vi "Teleop - Motor Data Logger (SubVI).vi"(4 "% Output":dbl, 6 "Battery Voltage":dbl, 7 "Reset":bool, 8 "Current":dbl, 10 "Velocity (ticks/100ms)":dbl, 11 "Position (ticks)":dbl) -> (0 "was teleop?":bool=TRUE, 1 "Time                            Position                    Velocity (RPM)          Acceleration             Current                     % Output                 Battery Voltage":dbl[][](array[numeric]), 2 "Delta V":dbl, 3 "acceleration":u32)   [LabVIEW 2019]
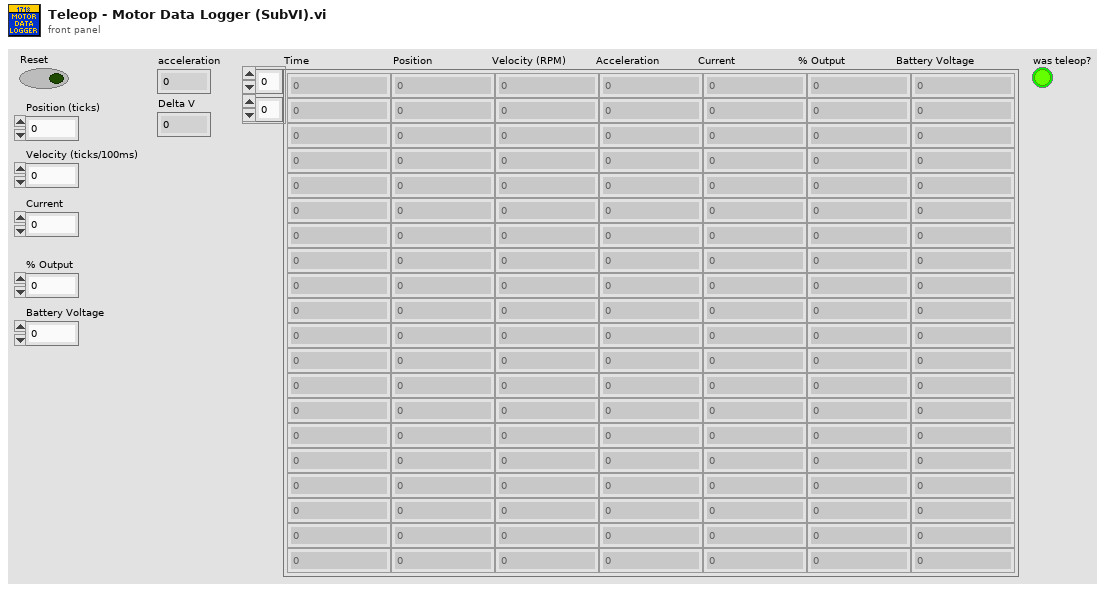
[diagram p1: front panel]
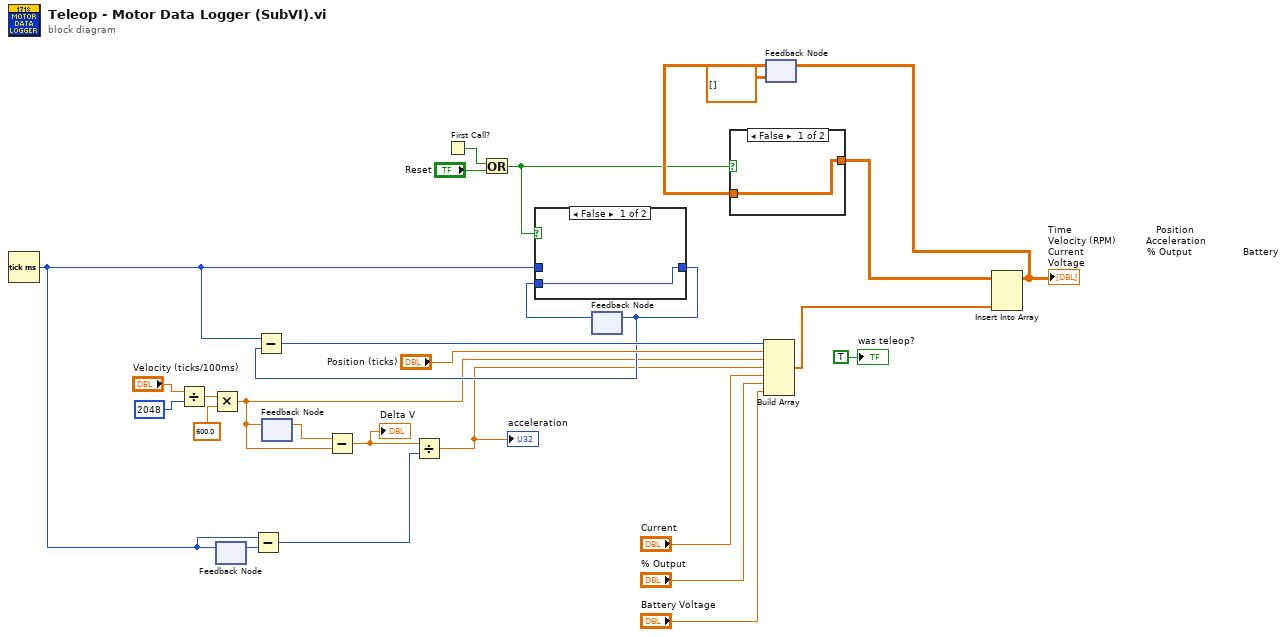
[diagram p0: block diagram]
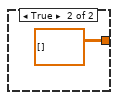
[diagram p3: hidden frame]
diagram:
  n1 = Tick Count (ms)() -> (millisecond timer value=w10:u32)
  n2 = Divide(x="Velocity (ticks/100ms)", y=2048) -> (x/y=w4:dbl)
  n3 = Multiply(x=w4, y=600.0) -> (x*y=w1:dbl)
  n4 = feedback-in #1(w10) -> ()
  n5 = feedback #1() -> (w11:u32)  [unwired: 1 in]
  n6 = Subtract(x=w10, y=w11) -> (x-y=w13:u32)
  n7 = feedback-in #2(w1) -> ()
  n8 = feedback #2() -> (w15:dbl)  [unwired: 1 in]
  n9 = Subtract(x=w15, y=w1) -> (x-y=w14:dbl)
  "Delta V" <- w14
  n10 = Divide(x=w14, y=w13) -> (x/y=w9:dbl)
  "acceleration" <- w9
  n11 = First Call?() -> (First Call?: T/F=w18:bool)
  n12 = Or(x=w18, y="Reset") -> (x .or. y?=w19:bool)
  n13 = feedback #3() -> (w21:u32)  [unwired: 1 in]
  n14 = case shown="False" w19 {
    tunnel: [w28 w29] -> w16
    tunnel: w10 -> [_ w29]
    tunnel: w21 -> [w28 _]
    frame False {
    }
    frame True {
    }
  }
  n15 = Subtract(x=w10, y=w16) -> (x-y=w20:u32)
  n16 = feedback-in #3(w16) -> ()
  n17 = Build Array(w20, "Position (ticks)", w1, w9, "Current", "% Output", "Battery Voltage") -> (w23:dbl[])
  n18 = feedback #4(dbl[][] [] ("array")) -> (w27:dbl[][])
  n19 = case shown="False" w19 {
    tunnel: [w30 dbl[][] [] ("array")] -> w24
    tunnel: w27 -> [w30 _]
    frame False {
    }
    frame True {
    }
  }
  n20 = Insert Into Array(array=w24, new element=w23) -> (w22:dbl[][])  [unwired: 2 in]
  "Time                            Position                    Velocity (RPM)          Acceleration             Current                     % Output                 Battery Voltage" <- w22
  n21 = feedback-in #4(w22) -> ()
  "was teleop?" <- TRUE ("was teleop?")
